vi "Actor Core.vi"(8 "error in":errorcluster, 11 "ClientUI in":refnum<class "ClientUI.lvclass">) -> (0 "error out":errorcluster, 3 "Actor out":refnum<class "Actor.lvclass">)   [LabVIEW 2018, in "ClientUI.lvlib" / "ClientUI.lvclass"]
doc: "(<B>Filename</B>: Actor Framework.lvlib:Actor.lvclass:Actor Core.vi)\n\nReceives messages to the actor, reacts to them, and initiates any error handling that may shut the actor down.\n\nDescendant classes may override this VI to append parallel tasks for the actor to complete while it handles messages. Overrides use the Call Parent Method node."
uses:
  ClientUI.lvclass
  <vilib>/ActorFramework/Actor/Actor.lvclass
  ClientUI.lvclass/ClientUI.ctl
  TCP_Client/TCP_Client/TCP_Client.lvclass
panel:
  out "Waveform Graph":dbl[](graph)
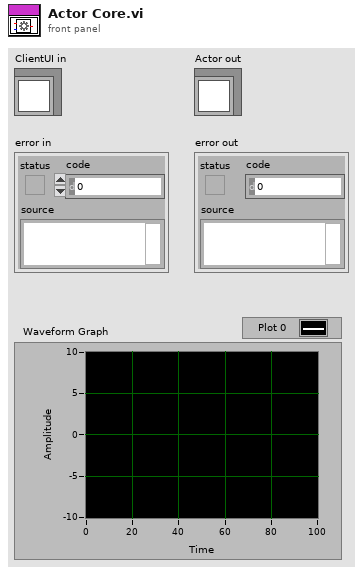
[diagram p1: front panel]
types:
  T1 = cluster{"stop":refnum<user-event>, "data":refnum<user-event>}
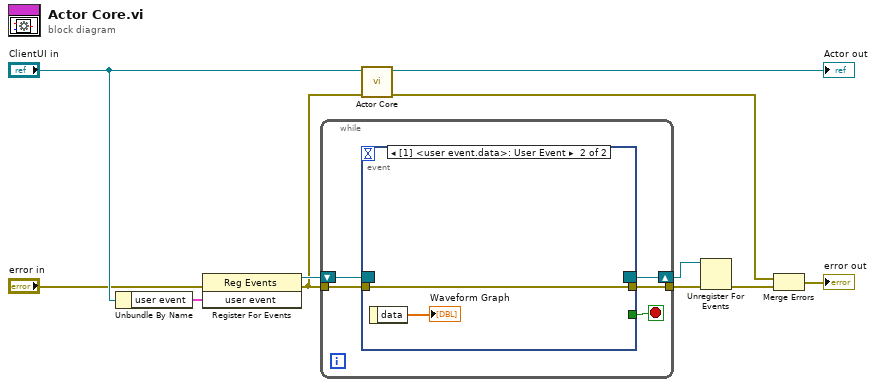
[diagram p0: block diagram]
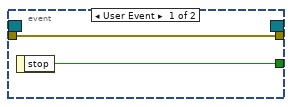
[diagram p2: hidden frame]
diagram:
  n1 = Unbundle By Name("ClientUI in") -> ("user event"=w8:T1)
  n2 = register-events(error in="error in", w8) -> (reference out=w6:refnum<event-registration>, error out=w5:errorcluster)  [unwired: 1 in]
  n3 = while {
    shift-right: [w13] -> w3
    shift-left: w6 -> [w16]
    tunnel: w5 -> [w15]
    tunnel: [w14] -> w4
    stop <- w12 stop-if-true
    n4 = event shown="[1] <user event.data>: User Event" {
      selector: w16 -> [_ _]
      dyn-events: [_ _] -> w13
      timeout: _ -> [_ _]
      tunnel: w15 -> [w18 w20]
      tunnel: [w18 w20] -> w14
      tunnel: [w17 _] -> w12
      event User Event {
        n5 = event-data() -> ("stop"=w17:bool)  [unwired: 1 in]
      }
      event User Event {
        n6 = event-data() -> ("data"=→"Waveform Graph":dbl[])  [unwired: 1 in]
      }
    }
  }
  n7 = call-parent "Actor Core.vi"("error in"=w5, "Actor in"="ClientUI in") -> ("error out"=w11:errorcluster, "Actor out"=→"Actor out":refnum<class "Actor.lvclass">)  [unwired: 8 in]
  n8 = Unregister For Events(event registration refnum=w3, error in=w4) -> (error out=w1:errorcluster)
  n9 = Merge Errors(w11, w1) -> (→"error out":errorcluster)
